vi "XMT-RCV Params.vi"(9 "Dig Channels":i32, 10 "Ann Array Params":T2={"Synth Foc?"=FALSE, "Focal Zones"=41, "Switch T/R"=0, "Trans Geometry (mm)"={"Transducer"=0, "Geo Focus"=12.0, "a (radius)"=3.0, "# of rings"=5, "kerf space "=0.1, "Center Freq"=12.0}, "Sub Ap Excite?"=FALSE, "Full Array Scan?"=FALSE, "Xmt/Rcv"={"XMIT"=[TRUE, TRUE, TRUE, TRUE, TRUE], "RCV"=[TRUE, TRUE, TRUE, TRUE, TRUE]}, "PulseSpacing (us)"=0.0, "Xmit Ring"=0, "XMIT CHS"=0, "RCV CHS"=0, "GPU?"=FALSE, "Save TIFF?"=FALSE, "downfactor"=1, "RCV 1CH"=0} {"RCV 1CH" items=["All", "1", "2", "3", "4", "5"]; "Trans Geometry (mm)"."Transducer" items=["6D 12R 40 MHz"=0, "10D 31R 20 MHz"=1, "10D 23R 20 MHz"=2, "6D 23R 40 MHz"=3, "4.5D 10.7R 40 MHz"=4, "9D 23.5R 20 MHz"=5, "9D 25.8R 20MHz"=6, "Enter"=99]; "Switch T/R" min=1 max=5 step=1}) -> (0 "GPU ordering":T1, 1 "# RCV":i16, 2 "# XMIT":i16, 3 "Recip Table":i16[][](array[numeric]), 4 "T/R String":string, 5 "virtual T/R count":i16)   [LabVIEW 2022 SP3]
uses:
  AnnularArray.ctl
  TransGeometry.ctl
  ArrayGeometry.ctl
  <vilib>/Analysis/baseanly.llb/Real Outer Product.vi
  <vilib>/Analysis/Matrix/Numeric/Conversions/Matrix To Array - RM.vi
  <vilib>/Analysis/NI_AALBase.lvlib
  <vilib>/Analysis/Matrix/NI_Matrix.lvlib
panel:
  out "ones weight":i16[](array[numeric])
  out "number of pairs":i32
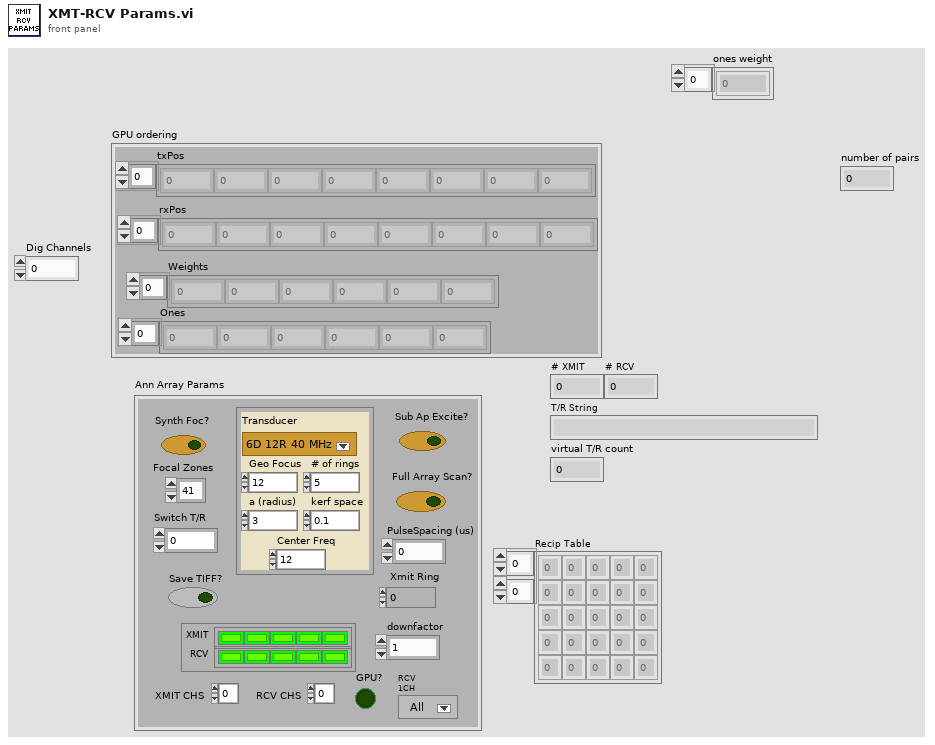
[diagram p1: front panel]
types:
  T1 = cluster{"txPos":i32[], "rxPos":i32[], "Weights":i16[], "Ones":i16[]}
  T2 = typedef "AnnularArray.ctl" = cluster{"Synth Foc?":bool, "Focal Zones":i16, "Switch T/R":i16, "Trans Geometry (mm)":T3, "Sub Ap Excite?":bool, "Full Array Scan?":bool, "Xmt/Rcv":cluster{"XMIT":bool[], "RCV":bool[]}, "PulseSpacing (us)":sgl, "Xmit Ring":i32, "XMIT CHS":u8, "RCV CHS":u8, "GPU?":bool, "Save TIFF?":bool, "downfactor":i32, "RCV 1CH":u16}
  T3 = typedef "TransGeometry.ctl" = cluster{"Transducer":T4, "Geo Focus":dbl, "a (radius)":dbl, "# of rings":i32, "kerf space ":dbl, "Center Freq":dbl}
  T4 = typedef "ArrayGeometry.ctl" = u16
  T5 = typedef "NI_Matrix.lvlib/RealMatrix.ctl" = dbl[][]
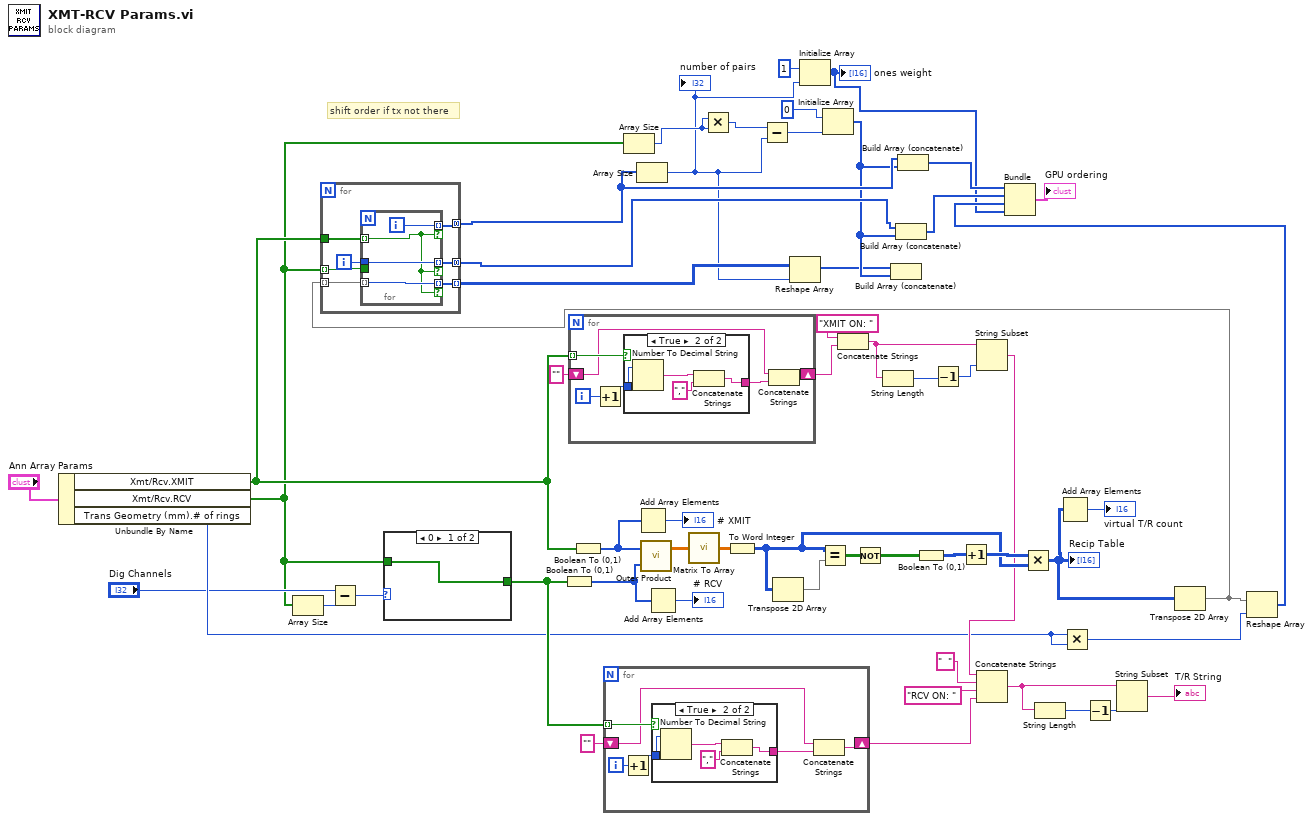
[diagram p0: block diagram]
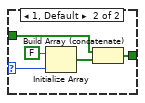
[diagram p2: hidden frame]
diagram:
  # "shift order if tx not there"
  n1 = Unbundle By Name("Ann Array Params") -> ("Xmt/Rcv.XMIT"=w19:bool[], "Xmt/Rcv.RCV"=w17:bool[], "Trans Geometry (mm).# of rings"=w22:i32)
  n2 = Array Size(array=w17) -> (size(s)=w28:i32)
  n3 = Subtract(x="Dig Channels", y=w28) -> (x-y=w27:i32)
  n4 = case shown="0" w27 {
    selector: w27 -> [_ w60]
    tunnel: w17 -> [w56 w59]
    tunnel: [w56 w57] -> w26
    frame 0 {
    }
    frame 1, Default {
      n5 = Initialize Array(FALSE ("Boolean"), w60) -> (w58:bool[])
      n6 = Build Array (concatenate)(w59, w58) -> (w57:bool[])
    }
  }
  n7 = Boolean To (0,1)(Boolean=w26) -> (0, 1=w47:i16[])
  n8 = for {
    tunnel: w19 -> [w67] mode=indexing
    shift-right: [w66] -> w43
    shift-left: "" -> [w62]
    i -> [w64]
    n9 = Increment(x=w64) -> (x+1=w63:i32)
    n10 = case shown="True" w67 {
      tunnel: w63 -> [_ w71]
      tunnel: [_ w69] -> w65
      frame False {
      }
      frame True {
        n11 = Number To Decimal String(number=w71) -> (decimal integer string=w70:string)  [unwired: 1 in]
        n12 = Concatenate Strings(w70, "," ("string")) -> (w69:string)
      }
    }
    n13 = Concatenate Strings(w62, w65) -> (w66:string)
  }
  n14 = Boolean To (0,1)(Boolean=w19) -> (0, 1=w48:i16[])
  n15 = for {
    tunnel: w26 -> [w77] mode=indexing
    shift-right: [w76] -> w40
    shift-left: "" -> [w72]
    i -> [w74]
    n16 = Increment(x=w74) -> (x+1=w73:i32)
    n17 = case shown="True" w77 {
      tunnel: w73 -> [_ w81]
      tunnel: [_ w79] -> w75
      frame False {
      }
      frame True {
        n18 = Number To Decimal String(number=w81) -> (decimal integer string=w80:string)  [unwired: 1 in]
        n19 = Concatenate Strings(w80, "," ("string")) -> (w79:string)
      }
    }
    n20 = Concatenate Strings(w72, w75) -> (w76:string)
  }
  n21 = Array Size(array=w17) -> (size(s)=w16:i32)
  n22 = Add Array Elements(numeric array=w48) -> (sum=→"# XMIT":i16)
  n23 = call-poly <vilib>:"Outer Product.vi"("Y Vector"=w47, "X Vector"=w48) -> ("Outer Product"=w55:T5)  [unwired: 1 out]
  n24 = Add Array Elements(numeric array=w47) -> (sum=→"# RCV":i16)
  n25 = call-poly <vilib>:"Matrix To Array.vi"("Real Matrix"=w55) -> ("Real 2D Array"=w50:dbl[][])
  n26 = Multiply(x=w16, y=w16) -> (x*y=w15:i32)
  n27 = To Word Integer(number=w50) -> (16bit integer=w49:i16[][])
  n28 = Transpose 2D Array(2D array=w49) -> (transposed array=w54:i16[][])
  n29 = Equal? ("Equal.vi")(x=w49, y=w54) -> (x = y?=w20:bool[][])
  n30 = Concatenate Strings("XMIT ON: " ("string"), w43) -> (w37:string)
  n31 = Not(x=w20) -> (.not. x?=w53:bool[][])
  n32 = String Length(string=w37) -> (length=w38:i32)
  n33 = Boolean To (0,1)(Boolean=w53) -> (0, 1=w52:i16[][])
  n34 = Decrement(x=w38) -> (x-1=w36:i32)
  n35 = Increment(x=w52) -> (x+1=w51:i16[][])
  n36 = String Subset(string=w37, length (rest)=w36) -> (substring=w35:string)  [unwired: 1 in]
  n37 = Concatenate Strings(w35, "  " ("string"), "RCV ON: " ("string"), w40) -> (w31:string)
  n38 = Multiply(x=w51, y=w49) -> (x*y=w25:i16[][])
  "Recip Table" <- w25
  n39 = String Length(string=w31) -> (length=w33:i32)
  n40 = Add Array Elements(numeric array=w25) -> (sum=→"virtual T/R count":i16)
  n41 = Multiply(x=w22, y=w22) -> (x*y=w23:i32)
  n42 = Decrement(x=w33) -> (x-1=w32:i32)
  n43 = String Subset(string=w31, length (rest)=w32) -> (substring=→"T/R String":string)  [unwired: 1 in]
  n44 = Transpose 2D Array(2D array=w25) -> (transposed array=w8:i16[][])
  n45 = for {
    tunnel: [w88] -> w11 mode=concatenating
    tunnel: [w86] -> w12 mode=concatenating
    tunnel: w19 -> [w84]
    tunnel: w17 -> [w85] mode=indexing
    tunnel: w8 -> [w83] mode=indexing
    tunnel: [w82] -> w5 mode=indexing
    i -> [w87]
    n46 = for {
      tunnel: [w92] -> w88 mode=indexing if=w89
      tunnel: w87 -> [w91]
      tunnel: [w91] -> w86 mode=indexing if=w89
      tunnel: w85 -> [_]
      tunnel: w84 -> [w89] mode=indexing
      tunnel: [w90] -> w82 mode=indexing if=w89
      tunnel: w83 -> [w90] mode=indexing
      i -> [w92]
    }
  }
  n47 = Array Size(array=w11) -> (size(s)=w3:i32)
  "number of pairs" <- w3
  n48 = Subtract(x=w15, y=w3) -> (x-y=w14:i32)
  n49 = Reshape Array(w5, w3) -> (w6:i16[])
  n50 = Initialize Array(i16 1 ("element"), w3) -> (w1:i16[])
  "ones weight" <- w1
  n51 = Initialize Array(0, w14) -> (w7:i32[])
  n52 = Build Array (concatenate)(w6, w7) -> ()  [unwired: 1 out]
  n53 = Build Array (concatenate)(w12, w7) -> (w9:i32[])
  n54 = Build Array (concatenate)(w11, w7) -> (w10:i32[])
  n55 = Reshape Array(w8, w23) -> (w4:i16[])
  n56 = Bundle(w10, w9, w4, w1) -> (→"GPU ordering":cluster{i32[], i32[], i16[], i16[]})  [unwired: 1 in]
